vi "ReadPWM.vi"(11 "Wheel":T1(ring)) -> (3 "PWM Counters":cluster{"High":dbl, "Low":dbl})   [LabVIEW 2013]
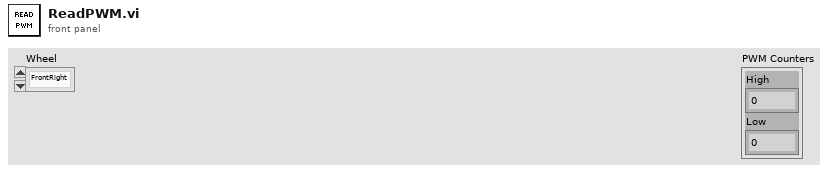
[diagram p1: front panel]
types:
  T1 = enum16{"FrontRight", "FrontLeft", "RearRight", "RearLeft"}
  T2 = typedef "WPI_CounterDevRef.ctl" = cluster{"DevStatus":errorcluster, "CntIndex":T3}
  T3 = typedef "FPGA_CounterCtrSystemIndex.ctl" = enum8{"Ctr 0", "Ctr 1", "Ctr 2", "Ctr 3", "Ctr 4", "Ctr 5", "Ctr 6", "Ctr 7", "Invalid"}
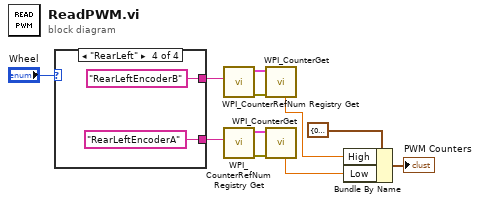
[diagram p0: block diagram]
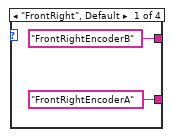
[diagram p2: hidden frame]
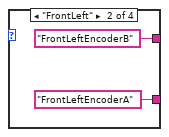
[diagram p3: hidden frame]
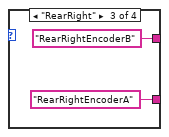
[diagram p4: hidden frame]
diagram:
  n1 = case shown="\"RearLeft\"" "Wheel" {
    tunnel: ["FrontRightEncoderA" "FrontLeftEncoderA" "RearRightEncoderA" "RearLeftEncoderA"] -> w8
    tunnel: ["FrontRightEncoderB" "FrontLeftEncoderB" "RearRightEncoderB" "RearLeftEncoderB"] -> w5
    frame "FrontRight", Default {
    }
    frame "FrontLeft" {
    }
    frame "RearRight" {
    }
    frame "RearLeft" {
    }
  }
  n2 = call <vilib>:"WPI_CounterRefNum Registry Get.vi"("refnum name"=w5) -> ("error out"=w6:errorcluster, "CounterDevRef"=w7:T2)  [unwired: 9 in]
  n3 = call <vilib>:"WPI_CounterRefNum Registry Get.vi"("refnum name"=w8) -> ("error out"=w10:errorcluster, "CounterDevRef"=w9:T2)  [unwired: 9 in]
  n4 = call <vilib>:"WPI_CounterGet.vi"("error in (no error)"=w6, "CounterDevRef in"=w7) -> ("Period (sec)"=w3:dbl)  [unwired: 4 in, 5 out]
  n5 = call <vilib>:"WPI_CounterGet.vi"("error in (no error)"=w10, "CounterDevRef in"=w9) -> ("Period (sec)"=w2:dbl)  [unwired: 4 in, 5 out]
  n6 = Bundle By Name(cluster=cluster{"High":dbl, "Low":dbl} {"High"=0.0, "Low"=0.0} ("PWM Counters"), "High"=w3, "Low"=w2) -> (→"PWM Counters":cluster{"High":dbl, "Low":dbl})
